vi "数据写入database.vi"(9 "data":variant, 10 "columns":string[](array[string]), 11 "table":string) -> (1 "error out":errorcluster)   [LabVIEW 2016, in "斯坦道CODMn.lvlib"]
uses:
  <vilib>/Utility/sysdir.llb/System Directory Type.ctl
  <vilib>/addons/database/Connection.llb/DB Tools Open Connec (String).vi
  <vilib>/addons/database/Connection.llb/Conn Execute.vi
  <vilib>/addons/database/Recordset.llb/Rec Fetch Recordset Data (R).vi
  <vilib>/addons/database/Recordset.llb/Rec Destroy - Connection.vi
  <vilib>/addons/database/NI_Database_API.lvlib
panel:
  out "为空？":bool
  out "recordset data":variant[][](array[variant])
  in  "error in (no error)":errorcluster
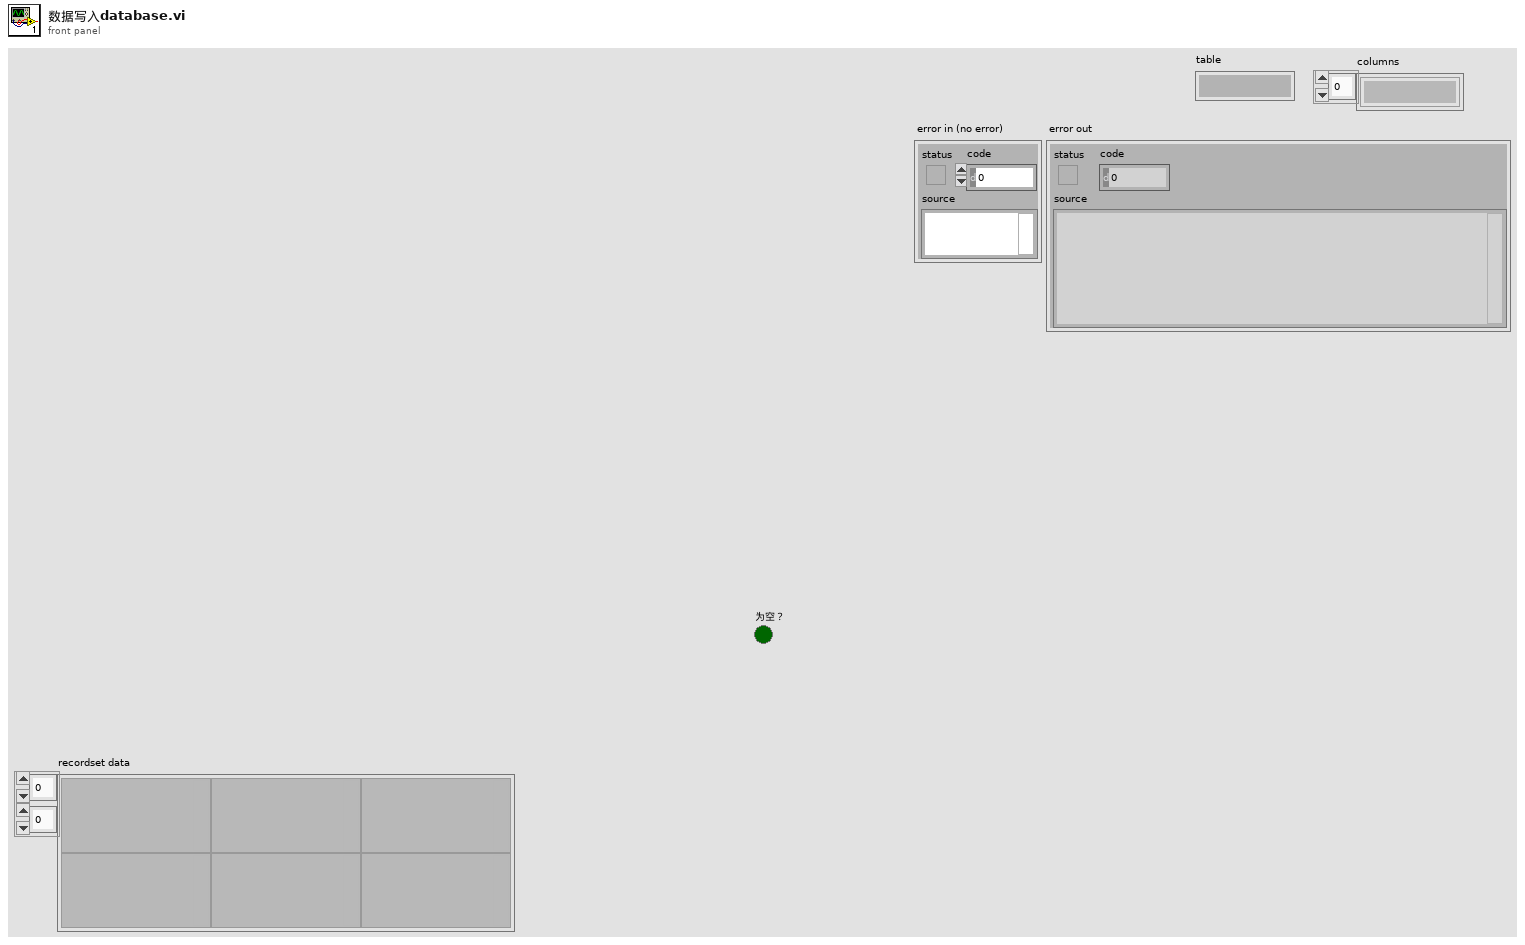
[diagram p1: front panel]
types:
  T1 = cluster{"时间":timestamp, "测量模式":string, "数据类型":string, "检测值":sgl, "单位":string, "数据标识":string, "因子编码":string, "标样参考值":sgl, "ORP-A":sgl, "ORP-B":sgl, "ORP-K":sgl, "COD滴定值":sgl, "高锰酸钾滴定数":sgl, "温度":sgl}
  T2 = typedef "System Directory Type.ctl" = i32
  T3 = typedef "NI_Database_API.lvlib/Conn ObjectReference.ctl" = refnum<k1>
  T4 = typedef "NI_Database_API.lvlib/Rec ObjectReference.ctl" = refnum<k1>
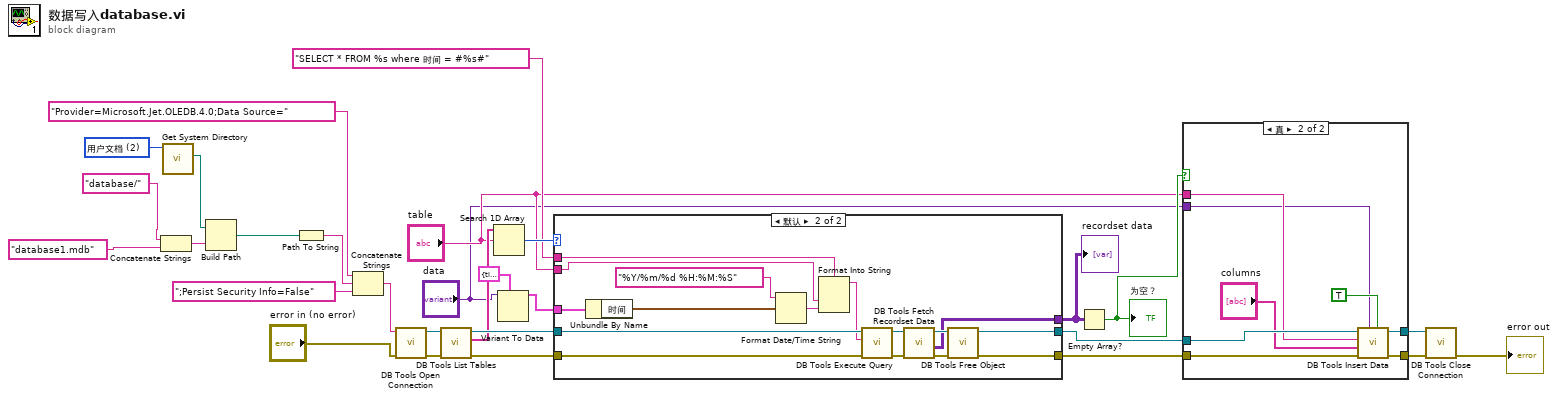
[diagram p0: block diagram]
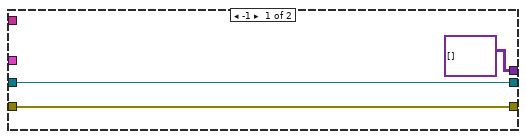
[diagram p3: hidden frame]
diagram:
  w29 = T2 2 items=["用户目录"=0, "用户桌面"=1, "用户文档"=2, "用户应用程序数据"=3, "用户设置"=4, "用户临时目录"=5, "公共文档"=6, "公共应用程序数据"=7, "公共设置"=8, "公共缓存"=13, "系统核心库"=9, "系统安装库"=10, "应用程序文件"=11, "启动盘根目录"=12] ("system directory type")
  n1 = Concatenate Strings("database/" ("condition"), "database1.mdb" ("字符串")) -> (w27:string)
  n2 = call <vilib>:"Get System Directory.vi"("system directory type"=w29) -> ("system directory"=w28:path)  [unwired: 10 in]
  n3 = Build Path(base path=w28, name or relative path=w27) -> (appended path=w1:path)
  n4 = Path To String(path=w1) -> (string=w23:string)
  n5 = Concatenate Strings("Provider=Microsoft.Jet.OLEDB.4.0;Data Source=" ("condition"), w23, ";Persist Security Info=False" ("condition")) -> (w21:string)
  n6 = call-poly <vilib>:"DB Tools Open Connection.vi"("error in (no error)"="error in (no error)", "connection information"=w21) -> ("error out"=w18:errorcluster, "connection reference"=w19:T3)  [unwired: 6 in]
  n7 = call <vilib>:"DB Tools List Tables.vi"("error in (no error)"=w18, "connection reference"=w19) -> ("error out"=w16:errorcluster, "tables"=w15:string[], "connection reference out"=w17:T3)  [unwired: 3 in]
  n8 = Search 1D Array(1D array=w15, element="table") -> (index of element=w14:i32)  [unwired: 1 in]
  n9 = Variant To Data(type=T1 {"时间"=timestamp(0 s since 1904-01-01), "测量模式"="", "数据类型"="", "检测值"=0.0, "单位"="", "数据标识"="", "因子编码"="", "标样参考值"=0.0, "ORP-A"=0.0, "ORP-B"=0.0, "ORP-K"=0.0, "COD滴定值"=0.0, "高锰酸钾滴定数"=0.0, "温度"=0.0} ("data"), Variant="data") -> (data=w3:T1)  [unwired: 1 in, 1 out]
  n10 = case shown="默认" w14 {
    tunnel: [variant[][] [] ("recordset data") w44] -> w20
    tunnel: [w32 w43] -> w10
    tunnel: [w31 w42] -> w11
    tunnel: w17 -> [w32 w41]
    tunnel: w16 -> [w31 w40]
    tunnel: "table" -> [_ w39]
    tunnel: "SELECT * FROM %s where 时间 = #%s#" ("格式字符串") -> [_ w38]
    tunnel: w3 -> [_ w33]
    frame -1 {
    }
    frame Default {
      n11 = Unbundle By Name(w33) -> ("时间"=w36:timestamp)
      n12 = Format Date/Time String(time format string (%c)="%Y/%m/%d %H:%M:%S" ("时间格式字符串(%c)"), seconds (now)=w36) -> (date/time string=w34:string)  [unwired: 1 in]
      n13 = Format Into String(format string=w38, w39, w34) -> (resulting string=w37:string)  [unwired: 2 in, 1 out]
      n14 = call-poly <vilib>:"DB Tools Execute Query.vi"("error in (no error)"=w40, "SQL query"=w37, "connection reference"=w41) -> ("error out"=w45:errorcluster, "recordset reference"=w48:T4)  [unwired: 5 in]
      n15 = call-poly <vilib>:"DB Tools Fetch Recordset Data.vi"("error in (no error)"=w45, "recordset reference"=w48) -> ("error out"=w46:errorcluster, "recordset data"=w44:variant[][], "recordset reference out"=w47:T4)  [unwired: 3 in]
      n16 = call-poly <vilib>:"DB Tools Free Object.vi"("error in (no error)"=w46, "recordset reference"=w47) -> ("error out"=w42:errorcluster, "connection reference"=w43:T3)  [unwired: 8 in]
    }
  }
  "recordset data" <- w20
  n17 = Empty Array?(array=w20) -> (empty?=w12:bool)
  "为空？" <- w12
  n18 = case shown="真" w12 {
    tunnel: "table" -> [_ w53]
    tunnel: "data" -> [_ w51]
    tunnel: w11 -> [w49 w58]
    tunnel: w10 -> [w50 w57]
    tunnel: [w50 w55] -> w9
    tunnel: [w49 w54] -> w8
    frame False {
    }
    frame True {
      n19 = call <vilib>:"DB Tools Insert Data.vi"("create table? (F)"=TRUE, "data"=w51, "error in (no error)"=w58, "columns"="columns", "table"=w53, "connection reference"=w57) -> ("error out"=w54:errorcluster, "connection reference out"=w55:T3)  [unwired: 4 in]
    }
  }
  n20 = call <vilib>:"DB Tools Close Connection.vi"("error in (no error)"=w8, "connection reference"=w9) -> ("error out"=→"error out":errorcluster)  [unwired: 5 in]
